vi "_f_bronkhorstWriteManual.vi"(8 "error in (no error)":errorcluster) -> (0 "error out":errorcluster, 1 "Dispositivos":T1=[["3", "NO", "M0000013", "Air", "1", "ln/mn", "0", "0"], ["4", "NO", "M0000014", "Air", "1", "ln/mn", "0", "0"], ["5", "NO", "M0000015", "Air", "1", "ln/mn", "0", "0"], ["6", "NO", "M0000016", "Air", "1", "ln/mn", "0", "0"], ["7", "NO", "M0000017", "Air", "1", "ln/mn", "0", "0"], ["8", "NO", "M0000018", "Air", "1", "ln/mn", "0", "0"], ["9", "NO", "M0000019", "Air", "1", "ln/mn", "0", "0"], ["10", "NO", "M0000020", "Air", "1", "ln/mn", "0", "0"], ["11", "NO", "M0000021", "Air", "1", "ln/mn", "0", "0"]] caption="MassFlowControllers")   [LabVIEW 2013]
uses:
  serialBronkhorst/_s_TablaBronkhorst.ctl
  _f_BronkhorstModuleControl.ctl
  P2022 TB INCAR GLOBALES.vi
panel:
  in  "Cancel":bool
  in  "Write":bool
  in  "Setpoints":string[][](table)=[["3", "NO", "M0000013", "Air", "1", "ln/mn", "0", "0"], ["4", "NO", "M0000014", "Air", "1", "ln/mn", "0", "0"], ["5", "NO", "M0000015", "Air", "1", "ln/mn", "0", "0"], ["6", "NO", "M0000016", "Air", "1", "ln/mn", "0", "0"], ["7", "NO", "M0000017", "Air", "1", "ln/mn", "0", "0"], ["8", "NO", "M0000018", "Air", "1", "ln/mn", "0", "0"], ["9", "NO", "M0000019", "Air", "1", "ln/mn", "0", "0"], ["10", "NO", "M0000020", "Air", "1", "ln/mn", "0", "0"], ["11", "NO", "M0000021", "Air", "1", "ln/mn", "0", "0"]] caption="Nuevos valores"
  out "Enable(T)":bool=TRUE
  out "VISA Bronkhorst":refnum<visa-resource-name>
  in  "Delay Time (s)":dbl=0.1
  out "Num. of nodes":u32=6
  # "Nuevos flujos de gases (FLOWBUS)"
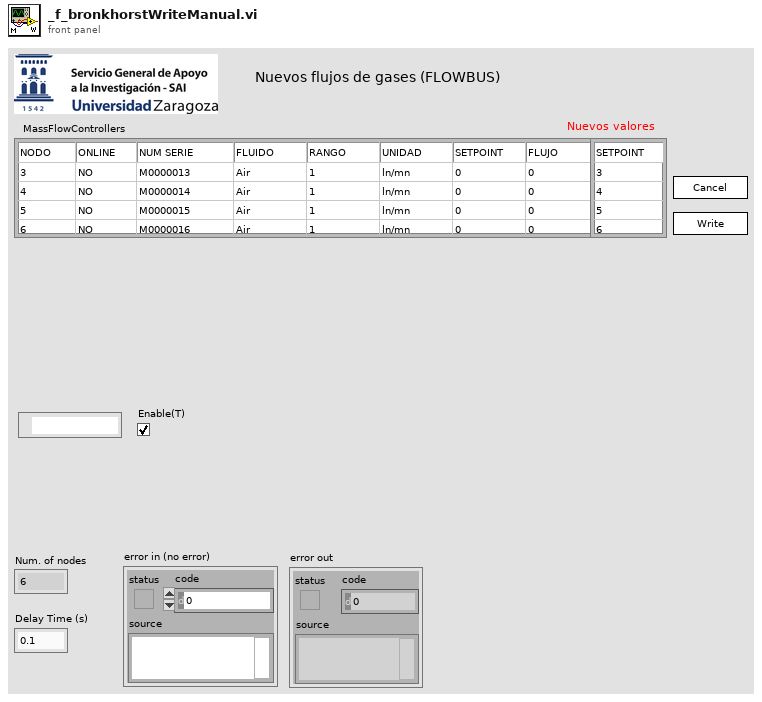
[diagram p1: front panel]
types:
  T1 = typedef "_s_TablaBronkhorst.ctl" = string[][]
  T2 = typedef "P2018 Bronkhorst Control.ctl" = cluster{"Dispositivos":T1, "NuevosSP":string[][], "Nodes":u32, "Delay(s)":dbl}
  T3 = typedef "P2018 Com Control.ctl" = cluster{"Flujo_1":refnum<visa-resource-name>, "Brk1":bool, "Flujo_2":refnum<visa-resource-name>, "Brk2":bool, "Flujo_3":refnum<visa-resource-name>, "Brk3":bool, "Flujo_4":refnum<visa-resource-name>, "Brk4":bool, "Eurothe":refnum<visa-resource-name>, "Eurot":bool, "Balanza":refnum<visa-resource-name>, "Bal":bool, "eValPos":refnum<visa-resource-name>, "eVal":bool, "flowbus":refnum<visa-resource-name>, "fb":bool}
  T4 = typedef "_f_BronkhorstModuleControl.ctl" = enum16{"RcharSerialNum", "RcharIdnString", "WuintFluidNum", "RuintFluidNum", "RcharFluidName", "RuintSensorType", "RfloatCap0", "RfloatCap100", "RcharCapUnitStr", "W%Setpoint", "R%Setpoint", "R%Measure", "WfloatSetpoint", "RfloatSetpoint", "RfloatMeasure ", "RfloatDensity", "WuintControlMode", "WcharRESET", "RfloatCounter", "RcharCounterUnit", "WfloatCounterLimit", "RfloatCounterLimit", "WcharCounterMode", "RcharCounterMode", "WcharCounterSPMode", "RcharCounterSPMode", "WcharCounterNewSP", "RcharCounterNewSP"}
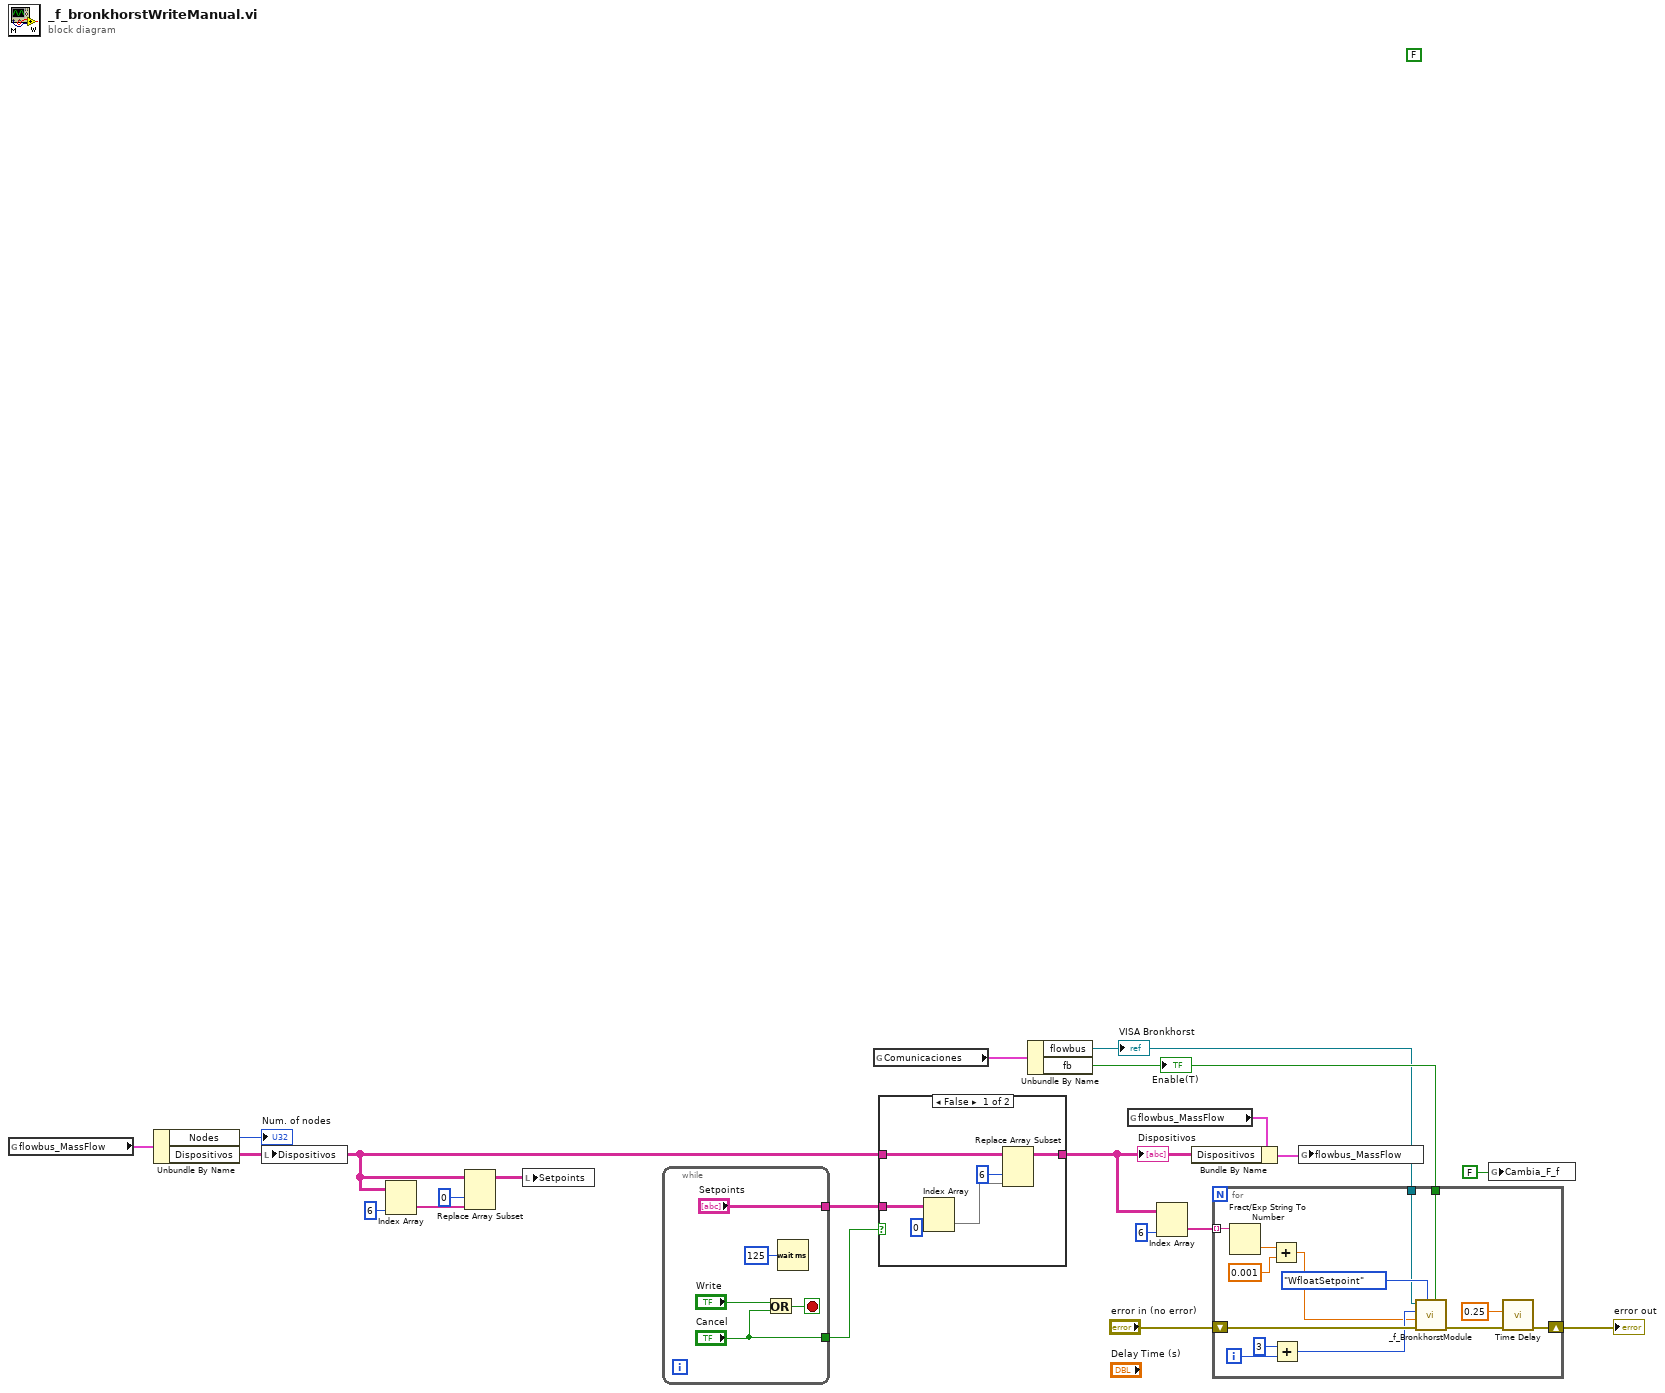
[diagram p0: block diagram]
diagram:
  (unwired) FALSE
  n1 = global read "P2022 TB INCAR GLOBALES.vi" "flowbus_MassFlow"() -> (w2:T2)
  n2 = Unbundle By Name(w2) -> ("Nodes"=→"Num. of nodes":u32, "Dispositivos"=w13:T1)
  n3 = local write "Dispositivos"(w13) -> ()
  n4 = Index Array(array=w13, index (col)=6 ("disabled index (col)")) -> (element=w16:string[])  [unwired: 1 in]
  n5 = Replace Array Subset(array=w13, new element=w16, index (col)=0 ("index")) -> (w17:T1)  [unwired: 1 in]
  n6 = local write "Setpoints"(w17) -> ()
  n7 = while {
    tunnel: ["Setpoints"] -> w14
    tunnel: ["Cancel"] -> w12
    stop <- w23 stop-if-true
    n8 = Or(x="Write", y="Cancel") -> (x .or. y?=w23:bool)
    n9 = Wait (ms)(milliseconds to wait=u32 125) -> ()  [unwired: 1 out]
  }
  n10 = global read "P2022 TB INCAR GLOBALES.vi" "Comunicaciones"() -> (w3:T3)
  n11 = case shown="False" w12 {
    tunnel: w14 -> [w28 _]
    tunnel: w13 -> [w27 w32]
    tunnel: [w26 w32] -> w8
    frame False {
      n12 = Index Array(array=w28, index (col)=0 ("disabled index (col)")) -> (element=w29:string[])  [unwired: 1 in]
      n13 = Replace Array Subset(array=w27, new element=w29, index (col)=6 ("index")) -> (w26:T1)  [unwired: 1 in]
    }
    frame True {
    }
  }
  "Dispositivos" <- w8
  n14 = Unbundle By Name(w3) -> ("flowbus"=w1:refnum<visa-resource-name>, "fb"=w6:bool)
  "Enable(T)" <- w6
  "VISA Bronkhorst" <- w1
  n15 = global read "P2022 TB INCAR GLOBALES.vi" "flowbus_MassFlow"() -> (w4:T2)
  n16 = Index Array(array=w8, index (col)=6 ("disabled index (col)")) -> (element=w7:string[])  [unwired: 1 in]
  n17 = Bundle By Name(cluster=w4, "Dispositivos"=w8) -> (w20:T2)
  n18 = for {
    shift-right: [w43] -> w10
    shift-left: "error in (no error)" -> [w46]
    tunnel: w7 -> [w38] mode=indexing
    tunnel: w6 -> [w34]
    tunnel: w1 -> [w33]
    i -> [w41]
    n19 = Fract/Exp String To Number(string=w38) -> (number=w37:dbl)  [unwired: 3 in, 1 out]
    n20 = Add(x=w37, y=0.001) -> (x+y=w36:dbl)
    n21 = Add(x=3, y=w41) -> (x+y=w40:i32)
    n22 = call "_f_BronkhorstModule.vi"("Enable(T)"=w34, "Command"=_f_BronkhorstModuleControl."WfloatSetpoint", "error in (no error)"=w46, "Value"=w36, "Nodo"=w40, "VISA resource name"=w33) -> ("error out"=w44:errorcluster)  [unwired: 2 in, 3 out]
    n23 = call "Time Delay"("error in (no error)"=w44, "Delay Time (s)"=0.25) -> ("error out"=w43:errorcluster)  [unwired: 9 in]
  }
  "error out" <- w10
  n24 = global write "P2022 TB INCAR GLOBALES.vi" "flowbus_MassFlow"(w20) -> ()
  n25 = global write "P2022 TB INCAR GLOBALES.vi" "Cambia_F_f"(FALSE ("ChangeF")) -> ()
